vi "read Kin v2.vi"(7 "file path":path) -> (0 "sensor 3 rotation":dbl[][](array[numeric]), 1 "sensor 1 rotation":dbl[][](array[numeric]), 2 "sensor 2 acceleration":dbl[][](array[numeric]), 3 "sensor 1 acceleration":dbl[][](array[numeric]), 4 "sensor 3 acceleration":dbl[][](array[numeric]), 5 "Frequency (Hz)":dbl, 6 "sensor 2 rotation":dbl[][](array[numeric]))   [LabVIEW 2009]
uses:
  <vilib>/Utility/file.llb/Read From Spreadsheet File (DBL).vi
panel:
  out "event":dbl[](array[numeric])
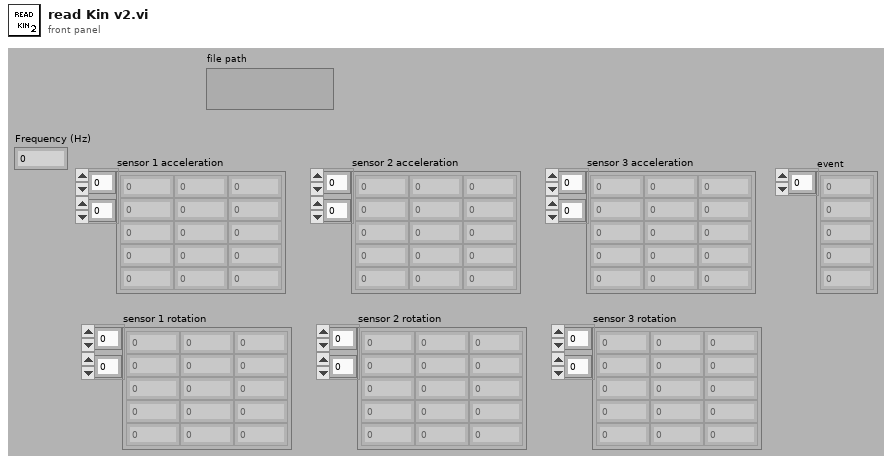
[diagram p1: front panel]
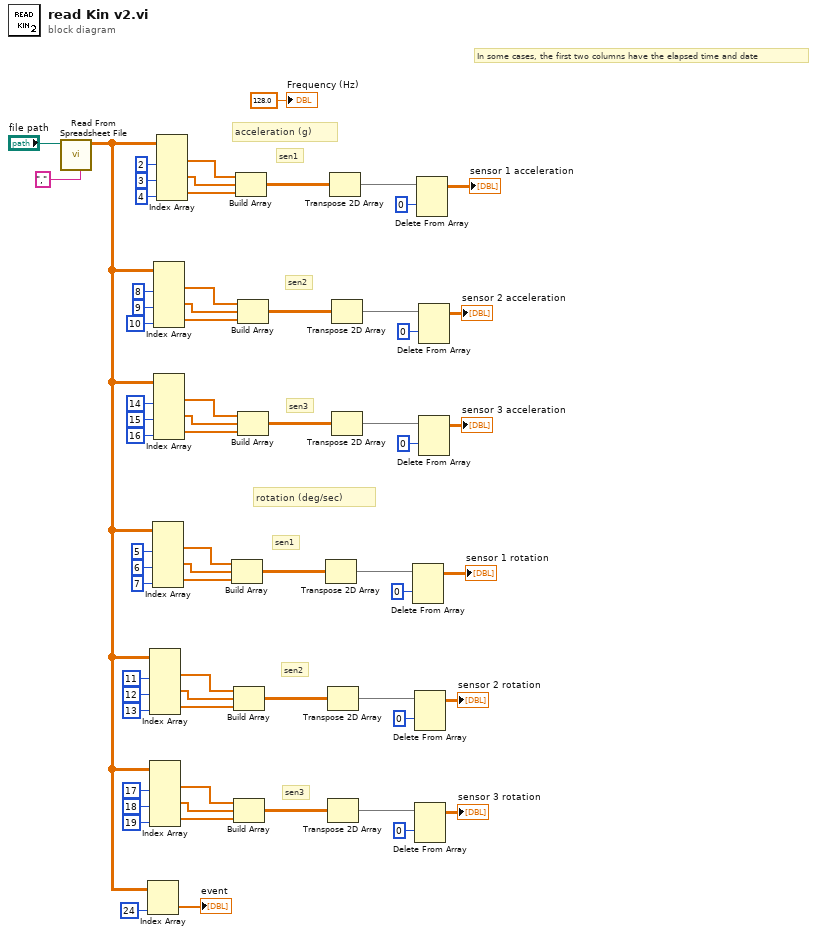
[diagram p0: block diagram]
diagram:
  # "In some cases, the first two columns have the elapsed time and date"
  # "sen3"
  # "sen2"
  # "sen1"
  # "rotation (deg/sec)"
  # "sen3"
  # "sen2"
  # "sen1"
  # "acceleration (g)"
  n1 = call-poly <vilib>:"Read From Spreadsheet File.vi"("delimiter (\\t)"="," ("delimiter (\\t)"), "file path (dialog if empty)"="file path") -> ("all rows"=w3:dbl[][])  [unwired: 5 in, 4 out]
  n2 = Index Array(array=w3, index (col)=24 ("disabled index (col)")) -> (element=→"event":dbl[])  [unwired: 1 in]
  n3 = Index Array(array=w3, index (col) #1=11 ("disabled index (col)"), index (col) #2=12 ("index (col)"), index (col) #3=13 ("index (col)")) -> (element #1=w17:dbl[], element #2=w18:dbl[], element #3=w19:dbl[])  [unwired: 3 in]
  n4 = Index Array(array=w3, index (col) #1=17 ("disabled index (col)"), index (col) #2=18 ("index (col)"), index (col) #3=19 ("index (col)")) -> (element #1=w7:dbl[], element #2=w8:dbl[], element #3=w9:dbl[])  [unwired: 3 in]
  n5 = Index Array(array=w3, index (col) #1=5 ("disabled index (col)"), index (col) #2=6 ("index (col)"), index (col) #3=7 ("index (col)")) -> (element #1=w31:dbl[], element #2=w30:dbl[], element #3=w29:dbl[])  [unwired: 3 in]
  n6 = Index Array(array=w3, index (col) #1=8 ("disabled index (col)"), index (col) #2=9 ("index (col)"), index (col) #3=10 ("index (col)")) -> (element #1=w48:dbl[], element #2=w49:dbl[], element #3=w50:dbl[])  [unwired: 3 in]
  n7 = Index Array(array=w3, index (col) #1=14 ("disabled index (col)"), index (col) #2=15 ("index (col)"), index (col) #3=16 ("index (col)")) -> (element #1=w38:dbl[], element #2=w39:dbl[], element #3=w40:dbl[])  [unwired: 3 in]
  n8 = Index Array(array=w3, index (col) #1=2 ("disabled index (col)"), index (col) #2=3 ("index (col)"), index (col) #3=4 ("index (col)")) -> (element #1=w62:dbl[], element #2=w61:dbl[], element #3=w60:dbl[])  [unwired: 3 in]
  n9 = Build Array(w31, w30, w29) -> (w28:dbl[][])
  n10 = Build Array(w17, w18, w19) -> (w22:dbl[][])
  n11 = Build Array(w7, w8, w9) -> (w12:dbl[][])
  n12 = Build Array(w62, w61, w60) -> (w59:dbl[][])
  n13 = Build Array(w48, w49, w50) -> (w53:dbl[][])
  n14 = Build Array(w38, w39, w40) -> (w43:dbl[][])
  n15 = Transpose 2D Array(2D array=w28) -> (transposed array=w27:dbl[][])
  n16 = Transpose 2D Array(2D array=w22) -> (transposed array=w21:dbl[][])
  n17 = Transpose 2D Array(2D array=w12) -> (transposed array=w11:dbl[][])
  n18 = Transpose 2D Array(2D array=w59) -> (transposed array=w58:dbl[][])
  n19 = Transpose 2D Array(2D array=w53) -> (transposed array=w52:dbl[][])
  n20 = Transpose 2D Array(2D array=w43) -> (transposed array=w42:dbl[][])
  n21 = Delete From Array(array=w27, index (row)=0) -> (array with subset deleted=→"sensor 1 rotation":dbl[][])  [unwired: 2 in, 1 out]
  n22 = Delete From Array(array=w21, index (row)=0) -> (array with subset deleted=→"sensor 2 rotation":dbl[][])  [unwired: 2 in, 1 out]
  n23 = Delete From Array(array=w11, index (row)=0) -> (array with subset deleted=→"sensor 3 rotation":dbl[][])  [unwired: 2 in, 1 out]
  n24 = Delete From Array(array=w58, index (row)=0) -> (array with subset deleted=→"sensor 1 acceleration":dbl[][])  [unwired: 2 in, 1 out]
  n25 = Delete From Array(array=w52, index (row)=0) -> (array with subset deleted=→"sensor 2 acceleration":dbl[][])  [unwired: 2 in, 1 out]
  n26 = Delete From Array(array=w42, index (row)=0) -> (array with subset deleted=→"sensor 3 acceleration":dbl[][])  [unwired: 2 in, 1 out]
  "Frequency (Hz)" <- 128.0 ("Frequency (Hz)")
